vi "Reactor Read Client.vi"() -> ()   [LabVIEW 2017]
uses:
  <vilib>/OPCUA/controls/NodeIds.ctl
  <vilib>/OPCUA/controls/NodeId.ctl
  <vilib>/OPCUA/NI OPC UA Client.lvlib
panel:
  in  "stop":bool
  out "error out":errorcluster
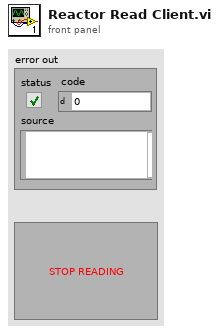
[diagram p1: front panel]
types:
  T1 = cluster{"message mode":enum16{"None", "Sign", "Sign and Encrypt"}, "security":enum16{"Basic256", "Basic128Rsa15"}}
  T2 = typedef "NodeIds.ctl" = T3[]
  T3 = typedef "NodeId.ctl" = string
  T4 = typedef "OPC UA Client Refnum.ctl" = refnum<k21>
  T5 = typedef "Subscription ID.ctl" = u32
  T6 = typedef "Subscription Data Change.ctl" = cluster{"node ID":T3, " value":variant, "timestamp":timestamp, "data type":T7, "status code":T8}
  T7 = typedef "Data Type.ctl" = u16
  T8 = typedef "OPC UA StatusCode.ctl" = u32
  T9 = cluster{"[0]":sgl, "[1]":sgl, "[2]":sgl, "[3]":sgl, "[4]":sgl, "[5]":sgl, "[6]":sgl, "[7]":sgl, "[8]":sgl, "[9]":sgl, "[10]":sgl, "[11]":sgl, "[12]":sgl, "[13]":sgl, "[14]":sgl, "[15]":sgl, "[16]":sgl, "[17]":sgl, "[18]":sgl, "[19]":sgl, "[20]":sgl, "[21]":sgl, "[22]":sgl, "[23]":sgl, "[24]":sgl, "[25]":sgl, "[26]":sgl, "[27]":sgl, "[28]":sgl, "[29]":sgl, "[30]":sgl, "[31]":sgl, "[32]":sgl, "[33]":sgl, "[34]":sgl, "[35]":sgl, "[36]":sgl, "[37]":sgl, "[38]":sgl, "[39]":sgl, "[40]":sgl, "[41]":sgl, "[42]":sgl, "[43]":sgl, "[44]":sgl, "[45]":sgl, "[46]":sgl, "[47]":sgl, "[48]":sgl, "[49]":sgl, "[50]":sgl, "[51]":sgl, "[52]":sgl, "[53]":sgl, "[54]":sgl, "[55]":sgl, "[56]":sgl, "[57]":sgl, "[58]":sgl, "[59]":sgl, "[60]":sgl, "[61]":sgl, "[62]":sgl}
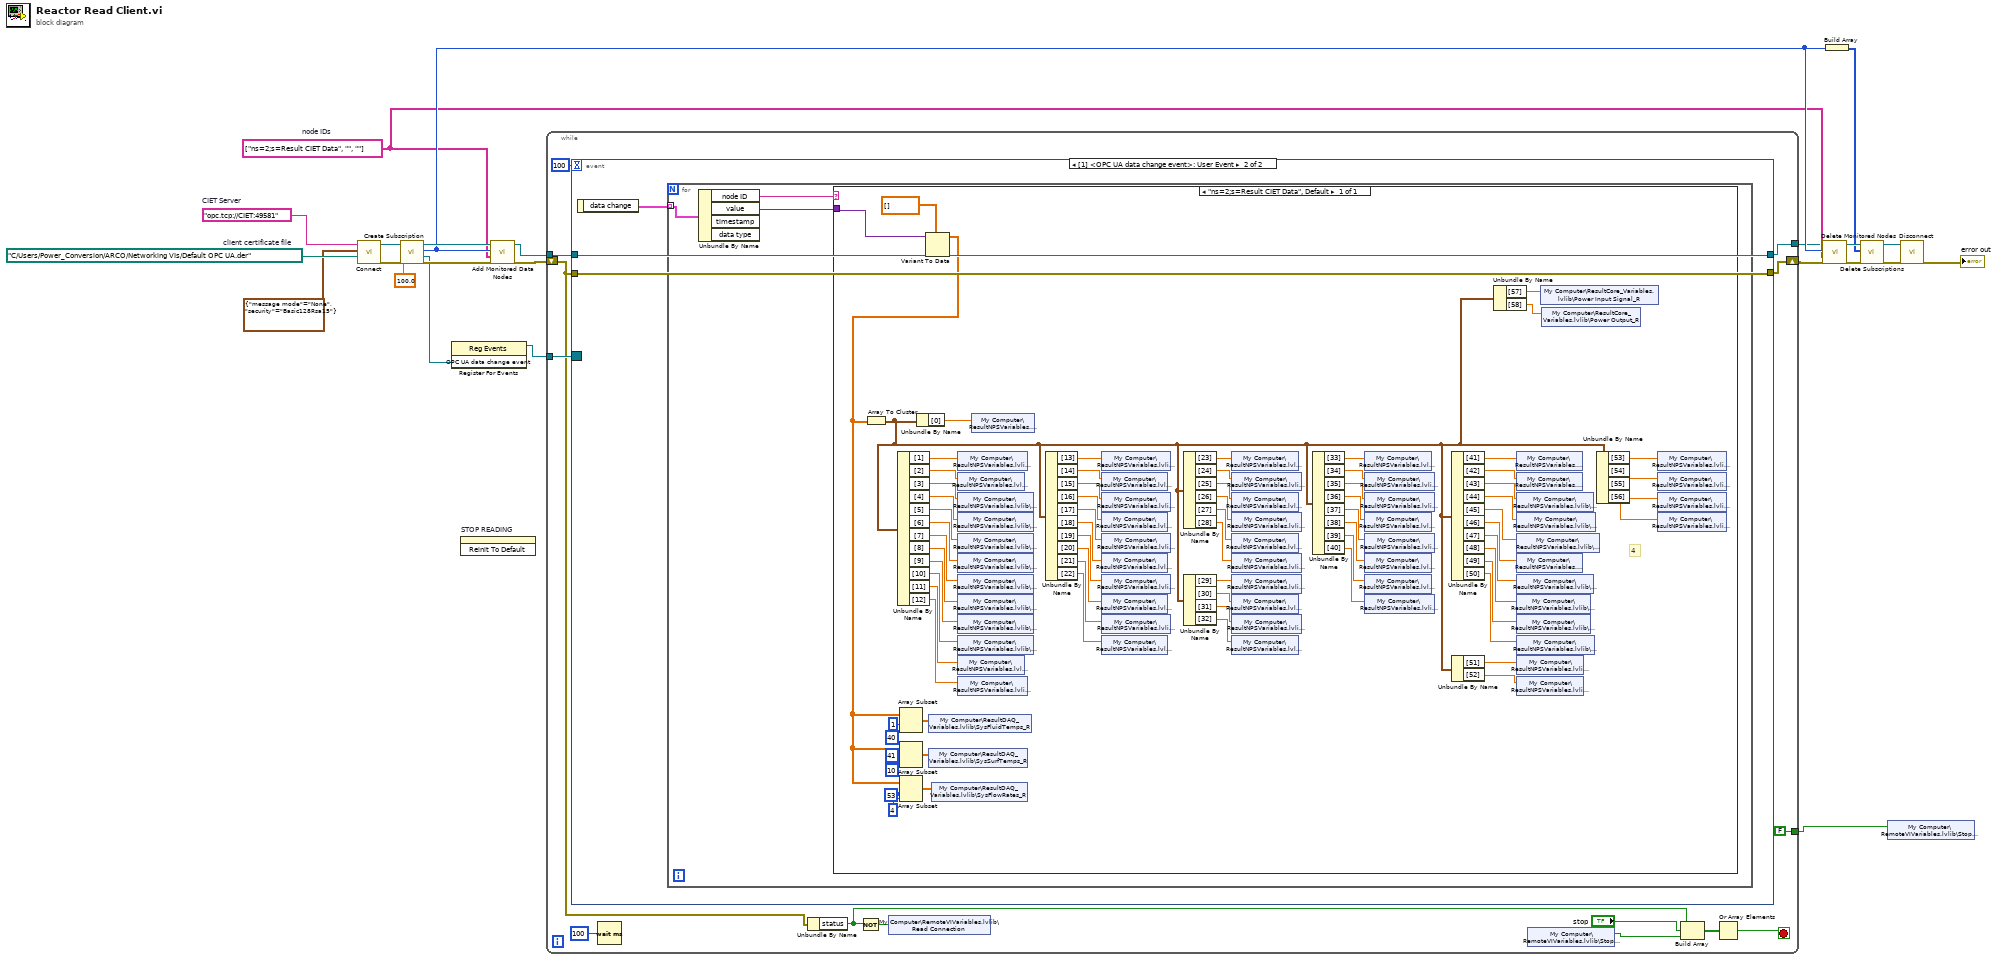
[diagram p0: block diagram]
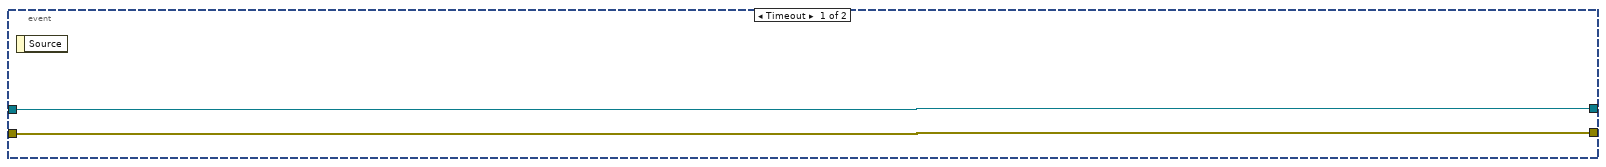
[diagram p2: hidden frame]
diagram:
  w6 = T2 ["ns=2;s=Result CIET Data", "", ""]  # node IDs
  w21 = path "C:/Users/Power_Conversion/ARCO/Networking VIs/Default OPC UA.der"  # client certificate file
  w22 = "opc.tcp://CIET:49581"  # CIET Server
  n1 = call <vilib>:"Connect.vi"("client certificate file"=w21, "security policy"=T1 {"message mode"=enum."None", "security"=enum."Basic128Rsa15"}, "server endpoint URL"=w22) -> ("error out"=w2:errorcluster, "OPC UA client refnum out"=w19:T4)  [unwired: 6 in, 1 out]
  n2 = call <vilib>:"Create Subscription.vi"("error in (no error)"=w2, "publishing interval (1000 ms)"=100.0, "OPC UA client refnum in"=w19) -> ("error out"=w17:errorcluster, "OPC UA data change event"=w16:refnum<user-event>, "subscription ID out"=w11:T5, "OPC UA client refnum out"=w18:T4)  [unwired: 4 in, 1 out]
  n3 = register-events(w16) -> (reference out=w9:refnum<event-registration>)  [unwired: 2 in, 1 out]
  n4 = invoke on="STOP READING" class="Bool" method="Reinit To Default"() -> ()  [unwired: 3 in, 3 out]
  n5 = call <vilib>:"Add Monitored Data Nodes.vi"("error in (no error)"=w17, "node IDs"=w6, "subscription ID in"=w11, "OPC UA client refnum in"=w18) -> ("error out"=w7:errorcluster, "OPC UA client refnum out"=w8:T4)  [unwired: 4 in, 2 out]
  n6 = while {
    tunnel: w9 -> [w37]
    tunnel: w8 -> [w36]
    tunnel: [w35] -> w5
    tunnel: [FALSE] -> w3
    shift-right: [w31] -> w1
    shift-left: w7 -> [w30]
    stop <- w29 stop-if-true
    n7 = event shown="[1] <OPC UA data change event>: User Event" {
      selector: w37 -> [_ _]
      dyn-events: _ -> [_ _]
      timeout: 100 -> [_ _]
      tunnel: w36 -> [w39 w42]
      tunnel: [w39 w42] -> w35
      tunnel: w30 -> [w38 w41]
      tunnel: [w38 w41] -> w31
      event Timeout {
        n8 = event-data() -> ()  [unwired: 1 in, 1 out]
      }
      event User Event {
        n9 = event-data() -> ("data change"=w40:T6[])  [unwired: 1 in]
        n10 = for {
          tunnel: w40 -> [w45] mode=indexing
          n11 = Unbundle By Name(w45) -> ("node ID"=w44:T3, "value"=w43:variant)  [unwired: 2 out]
          n12 = case shown="\"ns=2;s=Result CIET Data\", Default" w44 {
            tunnel: w43 -> [w51]
            frame "ns=2;s=Result CIET Data", Default {
              # "4"
              n13 = Variant To Data(type=sgl[] [], Variant=w51) -> (data=w50:sgl[])  [unwired: 1 in, 1 out]
              n14 = Array To Cluster(array=w50) -> (cluster=w48:T9)
              n15 = Unbundle By Name(w48) -> ("[1]"=w58:sgl, "[2]"=w60:sgl, "[3]"=w61:sgl, "[4]"=w62:sgl, "[5]"=w63:sgl, "[6]"=w64:sgl, "[7]"=w65:sgl, "[8]"=w66:sgl, "[9]"=w67:sgl, "[10]"=w68:sgl, "[11]"=w69:sgl, "[12]"=w70:sgl)
              n16 = Array Subset(array=w50, index=1, length=40) -> (w115:sgl[])
              n17 = Array Subset(array=w50, index=41, length=10) -> (w116:sgl[])
              n18 = Array Subset(array=w50, index=53, length=4) -> (w117:sgl[])
              n19 = Unbundle By Name(w48) -> ("[0]"=w59:sgl)
              n20 = shared-variable "My Computer\\ResultDAQ_Variables.lvlib\\SysFluidTemps_R"(w115) -> ()  [unwired: 1 in, 1 out]
              n21 = shared-variable "My Computer\\ResultDAQ_Variables.lvlib\\SysSurfTemps_R"(w116) -> ()  [unwired: 1 in, 1 out]
              n22 = shared-variable "My Computer\\ResultDAQ_Variables.lvlib\\SysFlowRates_R"(w117) -> ()  [unwired: 1 in, 1 out]
              n23 = shared-variable "My Computer\\ResultNPSVariables.lvlib\\WT-10_R"(w58) -> ()  [unwired: 1 in, 1 out]
              n24 = shared-variable "My Computer\\ResultNPSVariables.lvlib\\BT-11_R"(w60) -> ()  [unwired: 1 in, 1 out]
              n25 = shared-variable "My Computer\\ResultNPSVariables.lvlib\\CX-10-1_R"(w61) -> ()  [unwired: 1 in, 1 out]
              n26 = shared-variable "My Computer\\ResultNPSVariables.lvlib\\CX-10-2_R"(w62) -> ()  [unwired: 1 in, 1 out]
              n27 = shared-variable "My Computer\\ResultNPSVariables.lvlib\\CX-10-3_R"(w63) -> ()  [unwired: 1 in, 1 out]
              n28 = shared-variable "My Computer\\ResultNPSVariables.lvlib\\CX-10-4_R"(w64) -> ()  [unwired: 1 in, 1 out]
              n29 = shared-variable "My Computer\\ResultNPSVariables.lvlib\\CX-11-1_R"(w65) -> ()  [unwired: 1 in, 1 out]
              n30 = shared-variable "My Computer\\ResultNPSVariables.lvlib\\CX-11-2_R"(w66) -> ()  [unwired: 1 in, 1 out]
              n31 = shared-variable "My Computer\\ResultNPSVariables.lvlib\\CX-11-3_R"(w67) -> ()  [unwired: 1 in, 1 out]
              n32 = shared-variable "My Computer\\ResultNPSVariables.lvlib\\CX-11-4_R"(w68) -> ()  [unwired: 1 in, 1 out]
              n33 = shared-variable "My Computer\\ResultNPSVariables.lvlib\\BT-12_R"(w69) -> ()  [unwired: 1 in, 1 out]
              n34 = shared-variable "My Computer\\ResultNPSVariables.lvlib\\WT-13_R"(w70) -> ()  [unwired: 1 in, 1 out]
              n35 = shared-variable "My Computer\\ResultNPSVariables.lvlib\\Time_R"(w59) -> ()  [unwired: 1 in, 1 out]
              n36 = Unbundle By Name(w48) -> ("[13]"=w71:sgl, "[14]"=w72:sgl, "[15]"=w73:sgl, "[16]"=w74:sgl, "[17]"=w75:sgl, "[18]"=w76:sgl, "[19]"=w77:sgl, "[20]"=w78:sgl, "[21]"=w79:sgl, "[22]"=w80:sgl)
              n37 = shared-variable "My Computer\\ResultNPSVariables.lvlib\\WT-20_R"(w71) -> ()  [unwired: 1 in, 1 out]
              n38 = shared-variable "My Computer\\ResultNPSVariables.lvlib\\BT-21_R"(w72) -> ()  [unwired: 1 in, 1 out]
              n39 = shared-variable "My Computer\\ResultNPSVariables.lvlib\\WT-22_R"(w73) -> ()  [unwired: 1 in, 1 out]
              n40 = shared-variable "My Computer\\ResultNPSVariables.lvlib\\BT-23_R"(w74) -> ()  [unwired: 1 in, 1 out]
              n41 = shared-variable "My Computer\\ResultNPSVariables.lvlib\\WT-24_R"(w75) -> ()  [unwired: 1 in, 1 out]
              n42 = shared-variable "My Computer\\ResultNPSVariables.lvlib\\BT-25_R"(w76) -> ()  [unwired: 1 in, 1 out]
              n43 = shared-variable "My Computer\\ResultNPSVariables.lvlib\\WT-26_R"(w77) -> ()  [unwired: 1 in, 1 out]
              n44 = shared-variable "My Computer\\ResultNPSVariables.lvlib\\BT-27_R"(w78) -> ()  [unwired: 1 in, 1 out]
              n45 = shared-variable "My Computer\\ResultNPSVariables.lvlib\\WT-28_R"(w79) -> ()  [unwired: 1 in, 1 out]
              n46 = shared-variable "My Computer\\ResultNPSVariables.lvlib\\BT-29_R"(w80) -> ()  [unwired: 1 in, 1 out]
              n47 = Unbundle By Name(w48) -> ("[23]"=w81:sgl, "[24]"=w82:sgl, "[25]"=w83:sgl, "[26]"=w84:sgl, "[27]"=w85:sgl, "[28]"=w86:sgl)
              n48 = Unbundle By Name(w48) -> ("[29]"=w87:sgl, "[30]"=w88:sgl, "[31]"=w89:sgl, "[32]"=w90:sgl)
              n49 = shared-variable "My Computer\\ResultNPSVariables.lvlib\\BT-30_R"(w81) -> ()  [unwired: 1 in, 1 out]
              n50 = shared-variable "My Computer\\ResultNPSVariables.lvlib\\WT-31_R"(w82) -> ()  [unwired: 1 in, 1 out]
              n51 = shared-variable "My Computer\\ResultNPSVariables.lvlib\\BT-32_R"(w83) -> ()  [unwired: 1 in, 1 out]
              n52 = shared-variable "My Computer\\ResultNPSVariables.lvlib\\WT-33_R"(w84) -> ()  [unwired: 1 in, 1 out]
              n53 = shared-variable "My Computer\\ResultNPSVariables.lvlib\\BT-34_R"(w85) -> ()  [unwired: 1 in, 1 out]
              n54 = shared-variable "My Computer\\ResultNPSVariables.lvlib\\WT-35_R"(w86) -> ()  [unwired: 1 in, 1 out]
              n55 = shared-variable "My Computer\\ResultNPSVariables.lvlib\\WT-40_R"(w87) -> ()  [unwired: 1 in, 1 out]
              n56 = shared-variable "My Computer\\ResultNPSVariables.lvlib\\BT-41_R"(w88) -> ()  [unwired: 1 in, 1 out]
              n57 = shared-variable "My Computer\\ResultNPSVariables.lvlib\\WT-42_R"(w89) -> ()  [unwired: 1 in, 1 out]
              n58 = shared-variable "My Computer\\ResultNPSVariables.lvlib\\BT-43_R"(w90) -> ()  [unwired: 1 in, 1 out]
              n59 = Unbundle By Name(w48) -> ("[33]"=w91:sgl, "[34]"=w92:sgl, "[35]"=w93:sgl, "[36]"=w94:sgl, "[37]"=w95:sgl, "[38]"=w96:sgl, "[39]"=w97:sgl, "[40]"=w98:sgl)
              n60 = shared-variable "My Computer\\ResultNPSVariables.lvlib\\BT-60_R"(w91) -> ()  [unwired: 1 in, 1 out]
              n61 = shared-variable "My Computer\\ResultNPSVariables.lvlib\\WT-61_R"(w92) -> ()  [unwired: 1 in, 1 out]
              n62 = shared-variable "My Computer\\ResultNPSVariables.lvlib\\WT-62_R"(w93) -> ()  [unwired: 1 in, 1 out]
              n63 = shared-variable "My Computer\\ResultNPSVariables.lvlib\\BT-63_R"(w94) -> ()  [unwired: 1 in, 1 out]
              n64 = shared-variable "My Computer\\ResultNPSVariables.lvlib\\WT-64_R"(w95) -> ()  [unwired: 1 in, 1 out]
              n65 = shared-variable "My Computer\\ResultNPSVariables.lvlib\\BT-65_R"(w96) -> ()  [unwired: 1 in, 1 out]
              n66 = shared-variable "My Computer\\ResultNPSVariables.lvlib\\BT-66_R"(w97) -> ()  [unwired: 1 in, 1 out]
              n67 = shared-variable "My Computer\\ResultNPSVariables.lvlib\\WT-67_R"(w98) -> ()  [unwired: 1 in, 1 out]
              n68 = Unbundle By Name(w48) -> ("[41]"=w99:sgl, "[42]"=w100:sgl, "[43]"=w101:sgl, "[44]"=w102:sgl, "[45]"=w103:sgl, "[46]"=w104:sgl, "[47]"=w105:sgl, "[48]"=w106:sgl, "[49]"=w107:sgl, "[50]"=w108:sgl)
              n69 = Unbundle By Name(w48) -> ("[51]"=w109:sgl, "[52]"=w110:sgl)
              n70 = Unbundle By Name(w48) -> ("[57]"=w47:sgl, "[58]"=w46:sgl)
              n71 = shared-variable "My Computer\\ResultNPSVariables.lvlib\\ST-10_R"(w99) -> ()  [unwired: 1 in, 1 out]
              n72 = shared-variable "My Computer\\ResultNPSVariables.lvlib\\ST-11_R"(w100) -> ()  [unwired: 1 in, 1 out]
              n73 = shared-variable "My Computer\\ResultNPSVariables.lvlib\\ST-12-N_R"(w101) -> ()  [unwired: 1 in, 1 out]
              n74 = shared-variable "My Computer\\ResultNPSVariables.lvlib\\ST-12-SE_R"(w102) -> ()  [unwired: 1 in, 1 out]
              n75 = shared-variable "My Computer\\ResultNPSVariables.lvlib\\ST-12-SW_R"(w103) -> ()  [unwired: 1 in, 1 out]
              n76 = shared-variable "My Computer\\ResultNPSVariables.lvlib\\ST-13_R"(w104) -> ()  [unwired: 1 in, 1 out]
              n77 = shared-variable "My Computer\\ResultNPSVariables.lvlib\\ST-14-N_R"(w105) -> ()  [unwired: 1 in, 1 out]
              n78 = shared-variable "My Computer\\ResultNPSVariables.lvlib\\ST-14-E_R"(w106) -> ()  [unwired: 1 in, 1 out]
              n79 = shared-variable "My Computer\\ResultNPSVariables.lvlib\\ST-14-S_R"(w107) -> ()  [unwired: 1 in, 1 out]
              n80 = shared-variable "My Computer\\ResultNPSVariables.lvlib\\ST-14-W_R"(w108) -> ()  [unwired: 1 in, 1 out]
              n81 = shared-variable "My Computer\\ResultNPSVariables.lvlib\\AT-01_R"(w109) -> ()  [unwired: 1 in, 1 out]
              n82 = shared-variable "My Computer\\ResultNPSVariables.lvlib\\AT-02_R"(w110) -> ()  [unwired: 1 in, 1 out]
              n83 = shared-variable "My Computer\\ResultCore_Variables.lvlib\\Power Input Signal_R"(w47) -> ()  [unwired: 1 in, 1 out]
              n84 = shared-variable "My Computer\\ResultCore_Variables.lvlib\\Power Output_R"(w46) -> ()  [unwired: 1 in, 1 out]
              n85 = Unbundle By Name(w48) -> ("[53]"=w111:sgl, "[54]"=w112:sgl, "[55]"=w113:sgl, "[56]"=w114:sgl)
              n86 = shared-variable "My Computer\\ResultNPSVariables.lvlib\\FM-20_R"(w111) -> ()  [unwired: 1 in, 1 out]
              n87 = shared-variable "My Computer\\ResultNPSVariables.lvlib\\FM-30_R"(w112) -> ()  [unwired: 1 in, 1 out]
              n88 = shared-variable "My Computer\\ResultNPSVariables.lvlib\\FM-40_R"(w113) -> ()  [unwired: 1 in, 1 out]
              n89 = shared-variable "My Computer\\ResultNPSVariables.lvlib\\FM-60_R"(w114) -> ()  [unwired: 1 in, 1 out]
            }
          }
        }
      }
    }
    n90 = Wait (ms)(milliseconds to wait=u32 100 ("millisecond timer value")) -> ()  [unwired: 1 out]
    n91 = Unbundle By Name(w30) -> ("status"=w25:bool)
    n92 = Not(x=w25) -> (.not. x?=w32:bool)
    n93 = shared-variable "My Computer\\RemoteVIVariables.lvlib\\Read Connection"(w32) -> ()  [unwired: 1 in, 1 out]
    n94 = shared-variable "My Computer\\RemoteVIVariables.lvlib\\Stop Reading"() -> (w28:bool)  [unwired: 1 in, 1 out]
    n95 = Build Array(w25, "stop", w28) -> (w26:bool[])
    n96 = Or Array Elements(Boolean array=w26) -> (logical OR=w29:bool)
  }
  n97 = call <vilib>:"Delete Monitored Nodes.vi"("error in (no error)"=w1, "node IDs"=w6, "subscription ID in"=w11, "OPC UA client refnum in"=w5) -> ("error out"=w12:errorcluster, "OPC UA client refnum out"=w13:T4)  [unwired: 3 in, 3 out]
  n98 = Build Array(w11) -> (w10:T5[])
  n99 = call <vilib>:"Delete Subscriptions.vi"("error in (no error)"=w12, "subscription IDs"=w10, "OPC UA client refnum in"=w13) -> ("error out"=w14:errorcluster, "OPC UA client refnum out"=w15:T4)  [unwired: 6 in, 1 out]
  n100 = shared-variable "My Computer\\RemoteVIVariables.lvlib\\Stop Reading"(w3) -> ()  [unwired: 1 in, 1 out]
  n101 = call <vilib>:"Disconnect.vi"("error in (no error)"=w14, "OPC UA client refnum in"=w15) -> ("error out"=→"error out":errorcluster)  [unwired: 9 in]
